vi "Write PreviousTagY.vi"(8 "error in (no error)":errorcluster, 10 "PreviousTagY":dbl, 11 "Tag in":refnum<class "Tag.lvclass">) -> (0 "error out":errorcluster, 3 "Tag out":refnum<class "Tag.lvclass">)   [LabVIEW 2014, in "Tag.lvclass"]
uses:
  Tag.lvclass
  Tag.lvclass/Tag.ctl
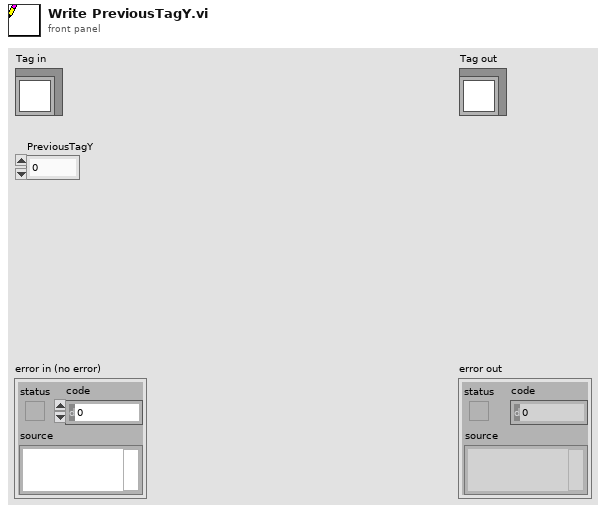
[diagram p1: front panel]
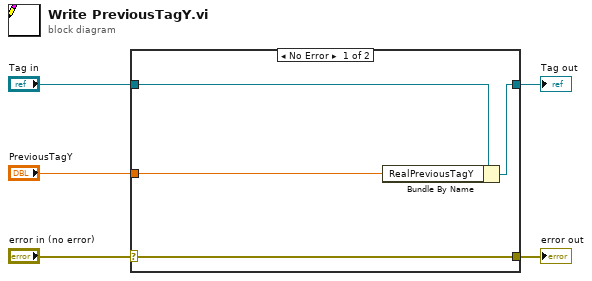
[diagram p0: block diagram]
diagram:
  n1 = case shown="No Error" "error in (no error)" {
    selector: "error in (no error)" -> [w9 w10]
    tunnel: [w9 w10] -> w4
    tunnel: [w7 w11] -> w2
    tunnel: "Tag in" -> [w8 w11]
    tunnel: "PreviousTagY" -> [w6 _]
    frame No Error {
      n2 = Bundle By Name(cluster=w8, "RealPreviousTagY"=w6) -> (w7:refnum<class "Tag.lvclass">)
    }
    frame Error {
    }
  }
  "error out" <- w4
  "Tag out" <- w2
